vi "Simulation4Updated.vi"() -> ()   [LabVIEW 2024]
panel:
  out "out":dbl
  in  "in":dbl
  in  "Python path":path
  in  "module path":path
  in  "function name":string
  out "A2P":bool(c317)
  out "Actuator Valve 2":bool
  out "A1P":bool(c317)
  in  "Actuator Valve 1":bool
  out "Multi-Segment Pipe 5":bool(c317)
  out "A2_pipe":bool(c317)
  out "A1_pipe":bool(c317)
  out "Multi-Segment Pipe 10":bool(c317)
  out "Multi-Segment Pipe 9":bool(c317)
  in  "stop":bool
  in  "Oil Pump":bool
  out "S2":bool
  out "S1":bool
  out "Tank 2":dbl(slide) scale=0.0..100.0
  out "Multi-Segment Pipe 7":bool(c317)
  out "Multi-Segment Pipe 6":bool(c317)
  out "Multi-Segment Pipe 4":bool(c317)
  out "Multi-Segment Pipe 3":bool(c317)
  out "Multi-Segment Pipe 2":bool(c317)
  out "Tank 1":dbl(slide) scale=0.0..100.0
  # "Level Sensor"
  # "Oil Source"
  # "Level Sensor"
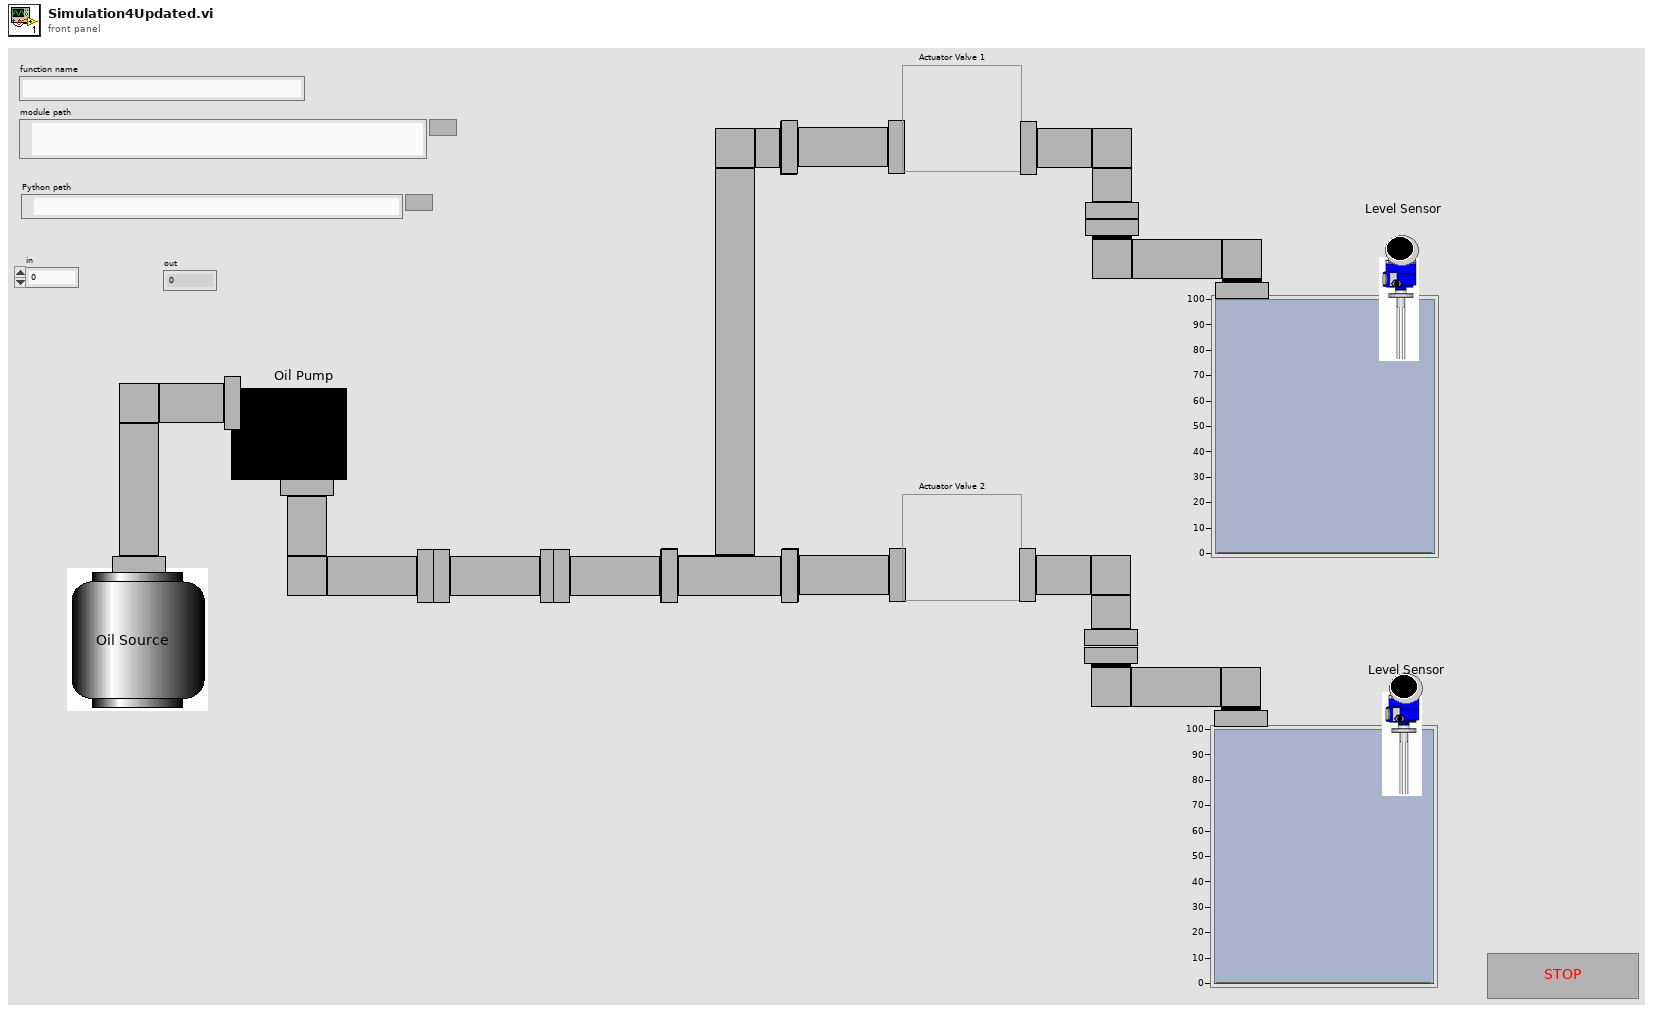
[diagram p1: front panel]
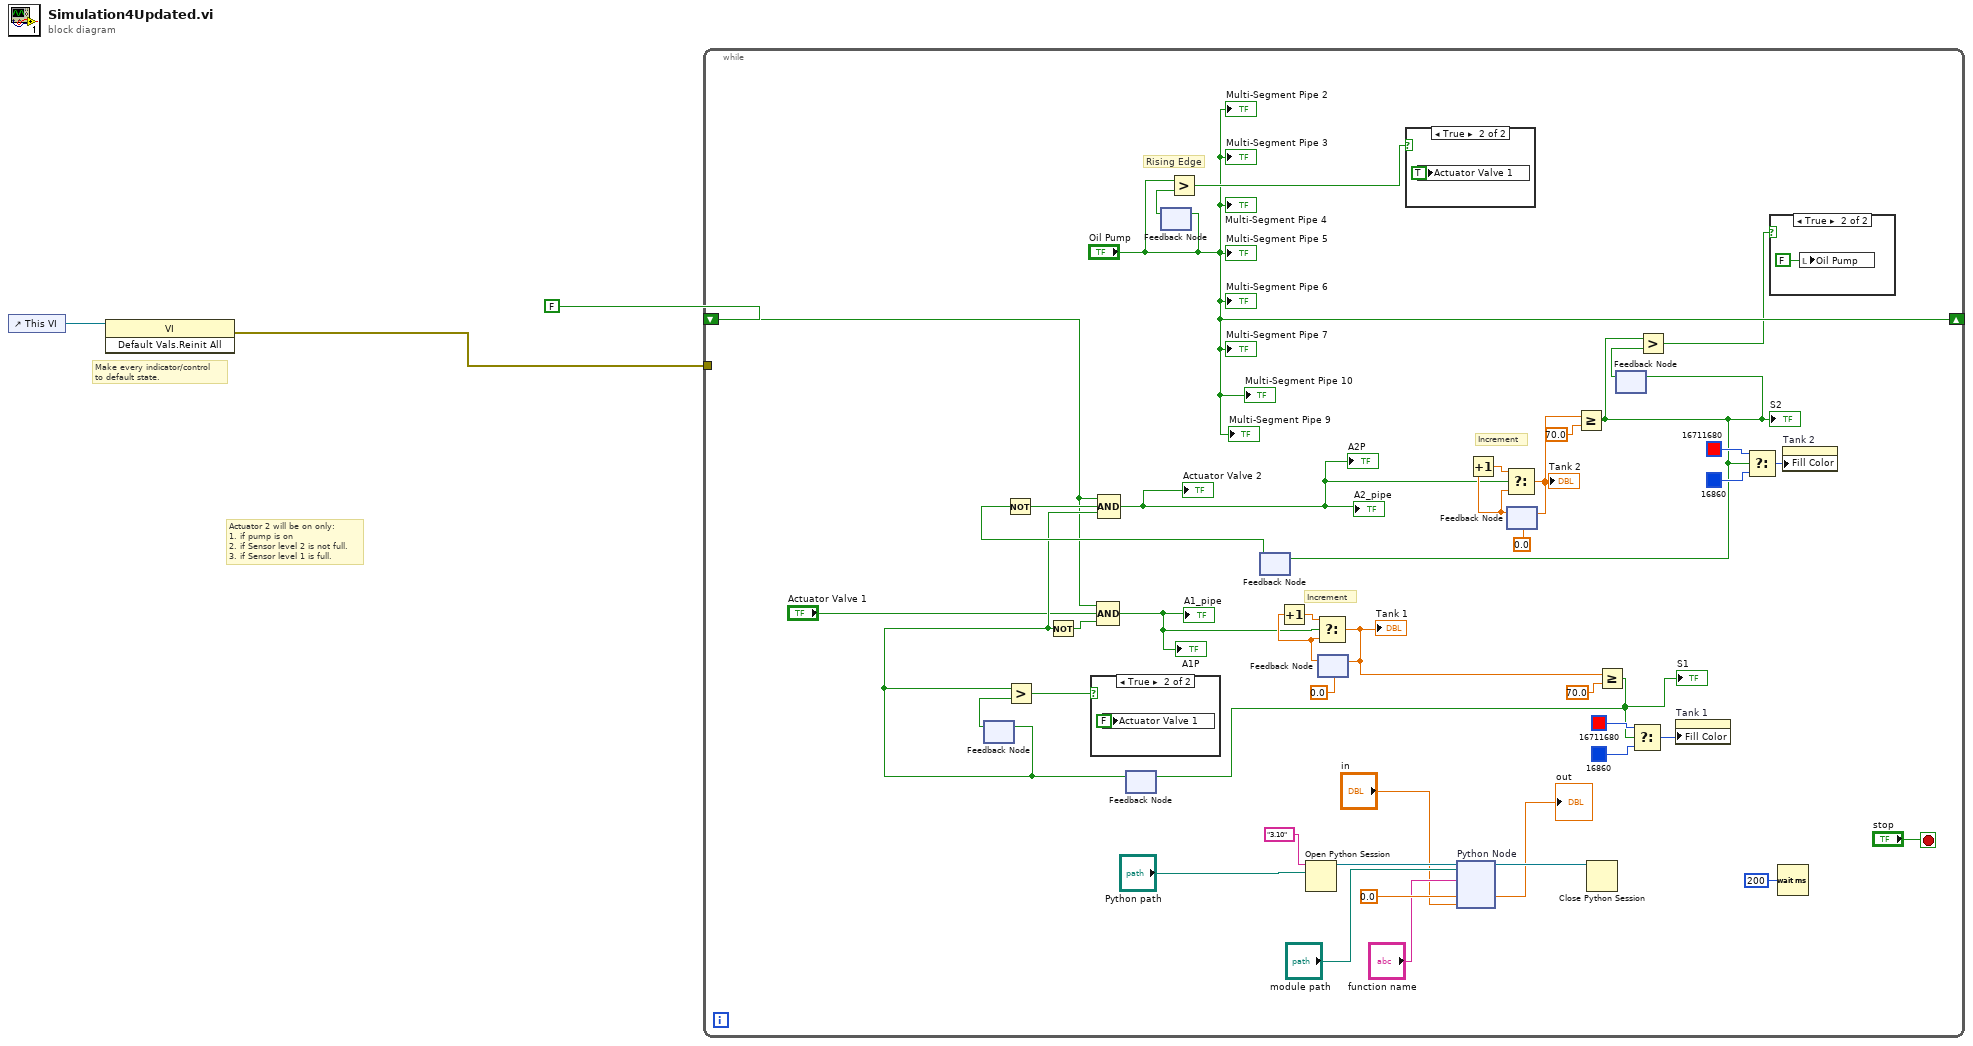
[diagram p0: block diagram]
diagram:
  # "Actuator 2 will be on only:\n1. if pump is on\n2. if Sensor level 2 is not full.\n3. if Sensor level 1 is full."
  # "Make every indicator/control\nto default state."
  n1 = control-ref of="This VI"() -> (w2:refnum<vi>)
  n2 = invoke class="VI" method="Default Vals.Reinit All"(reference=w2) -> (error out=w1:errorcluster)  [unwired: 2 in, 2 out]
  n3 = while {
    shift-right: ["Oil Pump"] -> _
    shift-left: FALSE -> [w16]
    tunnel: w1 -> [_]
    stop <- "stop" stop-if-true
    # "Increment"
    # "Increment"
    # "Rising Edge"
    n4 = feedback #1() -> (w31:bool)  [unwired: 1 in]
    n5 = feedback #2() -> (w19:bool)  [unwired: 1 in]
    n6 = feedback-in #1(w19) -> ()
    n7 = Greater?(x=w19, y=w31) -> (0:w30:bool)
    n8 = Not(x=w19) -> (.not. x?=w29:bool)
    n9 = case shown="True" w30 {
      frame False {
      }
      frame True {
        n10 = local write "Actuator Valve 1"(FALSE ("Actuator 1")) -> ()
      }
    }
    n11 = Compound Arithmetic op=AND(w16, "Actuator Valve 1", w29) -> (w23:bool)
    "A1_pipe" <- w23
    "A1P" <- w23
    n12 = feedback #3() -> (w27:bool)  [unwired: 1 in]
    n13 = feedback-in #3("Oil Pump") -> ()
    n14 = Greater?(x="Oil Pump", y=w27) -> (0:w26:bool)
    n15 = feedback #4() -> (w20:bool)  [unwired: 1 in]
    n16 = Not(x=w20) -> (.not. x?=w28:bool)
    n17 = Compound Arithmetic op=AND(w16, w28, w19) -> (w22:bool)
    "A2_pipe" <- w22
    "Actuator Valve 2" <- w22
    "A2P" <- w22
    n18 = Open Python Session(python version="3.10" ("Python version"), python path="Python path") -> (session out=w10:refnum<k35>)  [unwired: 1 in, 1 out]
    n19 = feedback #5(0.0) -> (w42:dbl)
    n20 = Increment(x=w42) -> (x+1=w41:dbl)
    n21 = Select(t=w41, s=w23, f=w42) -> (s? t:f=w5:dbl)
    "Tank 1" <- w5
    n22 = feedback-in #5(w5) -> ()
    n23 = case shown="True" w26 {
      frame False {
      }
      frame True {
        n24 = local write "Actuator Valve 1"(TRUE ("Actuator 1")) -> ()
      }
    }
    n25 = node "Python Node"(w10, "module path", "function name", 0.0, "in") -> (w9:refnum<k35>, →"out":dbl)  [unwired: 2 in, 3 out]
    n26 = feedback #6(0.0) -> (w43:dbl)
    n27 = Increment(x=w43) -> (x+1=w44:dbl)
    n28 = Select(t=w44, s=w22, f=w43) -> (s? t:f=w40:dbl)
    "Tank 2" <- w40
    n29 = feedback-in #6(w40) -> ()
    n30 = Greater Or Equal?(x=w40, y=70.0) -> (x >= y?=w17:bool)
    "S2" <- w17
    n31 = feedback-in #4(w17) -> ()
    n32 = Close Python Session(session in=w9) -> ()  [unwired: 1 in, 1 out]
    n33 = Greater Or Equal?(x=w5, y=70.0) -> (x >= y?=w7:bool)
    "S1" <- w7
    n34 = feedback-in #2(w7) -> ()
    n35 = feedback #7() -> (w24:bool)  [unwired: 1 in]
    n36 = feedback-in #7(w17) -> ()
    n37 = Select(t=u32 16711680 ("Fill Color"), s=w7, f=u32 16860 ("Fill Color")) -> (s? t:f=w32:u32)
    n38 = Greater?(x=w17, y=w24) -> (0:w21:bool)
    n39 = property on="Tank 1" class="Slide (strict)"("Fill Color"=w32) -> ()  [unwired: 2 in, 2 out]
    n40 = Select(t=u32 16711680 ("Fill Color"), s=w17, f=u32 16860 ("Fill Color")) -> (s? t:f=w36:u32)
    n41 = case shown="True" w21 {
      frame False {
      }
      frame True {
        n42 = local write "Oil Pump"(FALSE ("Actuator 1")) -> ()
      }
    }
    n43 = Wait (ms)(milliseconds to wait=u32 200) -> ()  [unwired: 1 out]
    n44 = property on="Tank 2" class="Slide (strict)"("Fill Color"=w36) -> ()  [unwired: 2 in, 2 out]
    "Multi-Segment Pipe 2" <- "Oil Pump"
    "Multi-Segment Pipe 3" <- "Oil Pump"
    "Multi-Segment Pipe 4" <- "Oil Pump"
    "Multi-Segment Pipe 5" <- "Oil Pump"
    "Multi-Segment Pipe 6" <- "Oil Pump"
    "Multi-Segment Pipe 7" <- "Oil Pump"
    "Multi-Segment Pipe 9" <- "Oil Pump"
    "Multi-Segment Pipe 10" <- "Oil Pump"
  }
